vi "TDMS Total Channel Length page.vi"(8 "error in (no error)":errorcluster, 11 "Node Ptr":T1 format="%.0x") -> (0 "error out":errorcluster)   [LabVIEW 2011, in "TDMS Custom Device.lvlib"]
uses:
  TDMS Custom Device.lvlib
  <vilib>/NI Veristand/Custom Device API/Custom Device Item Ref.ctl
  <vilib>/NI Veristand/Custom Device API/Custom Device API.lvlib
panel:
  out "Total Channel Length (elements)":u32
  in  "Header":cluster{"Section Name":string}={"Section Name"="TDMS Mode Channel Settings"}
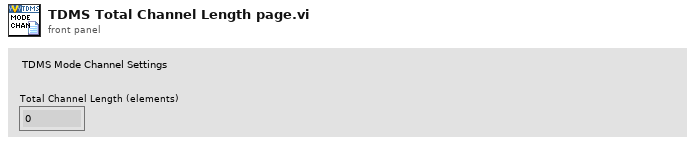
[diagram p1: front panel]
types:
  T1 = typedef "Custom Device API.lvlib/Custom Device Item Ref.ctl" = u64
  T2 = typedef "Custom Device API.lvlib/Custom Device Channel.ctl" = cluster{"Type":T3, "Units":string, "Default Value":dbl, "Faultable":bool, "Scalable":bool}
  T3 = typedef "Custom Device API.lvlib/Custom Device Channel Type.ctl" = enum16{"Input", "Output"}
  T4 = typedef "Custom Device API.lvlib/Custom Device Commands.ctl" = enum16{"Default", "Item renamed", "Shutdown", "Dynamic button pressed"}
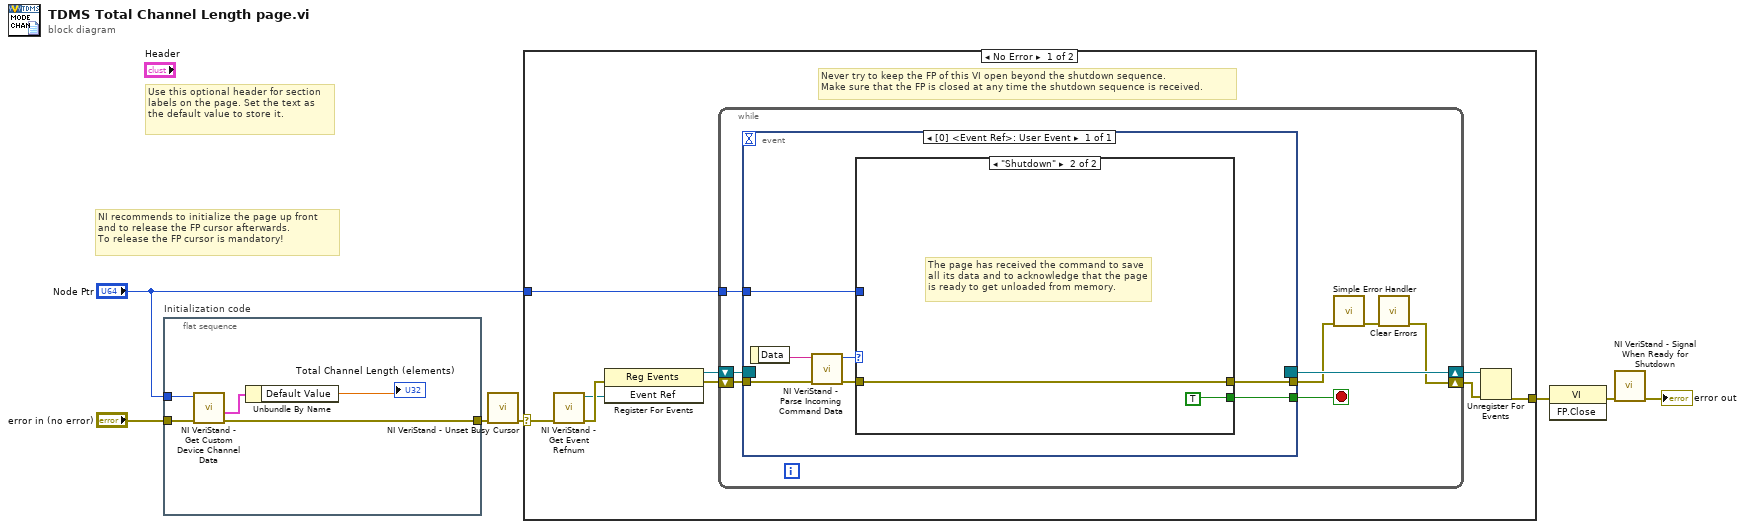
[diagram p0: block diagram]
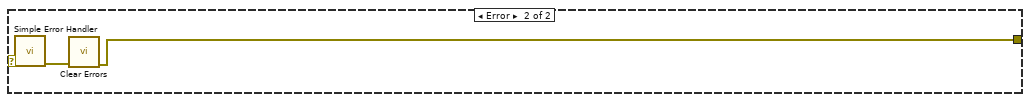
[diagram p3: hidden frame]
diagram:
  # "Use this optional header for section labels on the page. Set the text as the default value to store it."
  # "NI recommends to initialize the page up front\nand to release the FP cursor afterwards.\nTo release the FP cursor is mandatory!"
  n1 = flat-sequence "Initialization code" {
    tunnel: "error in (no error)" -> [w11]
    tunnel: "Node Ptr" -> [w10]
    tunnel: [w9] -> w1
    frame #0 {
      n2 = call <vilib>:"NI VeriStand - Get Custom Device Channel Data.vi"("error in (no error)"=w11, "Channel Ref in"=w10) -> ("error out"=w9:errorcluster, "Channel"=w12:T2)  [unwired: 8 out]
      n3 = Unbundle By Name(w12) -> ("Default Value"=→"Total Channel Length (elements)":dbl)
    }
  }
  n4 = call <vilib>:"NI VeriStand - Unset Busy Cursor.vi"("error in (no error)"=w1) -> ("error out"=w3:errorcluster)  [unwired: 10 out]
  n5 = case shown="No Error" w3 {
    selector: w3 -> [w13 w42]
    tunnel: [w18 w40] -> w7
    tunnel: "Node Ptr" -> [w14 _]
    frame No Error {
      # "Never try to keep the FP of this VI open beyond the shutdown sequence.\nMake sure that the FP is closed at any time the shutdown sequence is received."
      n6 = call <vilib>:"NI VeriStand - Get Event Refnum.vi"("error in (no error)"=w13) -> ("error out"=w21:errorcluster, "Event Ref"=w17:refnum<user-event>)  [unwired: 9 out]
      n7 = register-events(error in=w21, w17) -> (reference out=w15:refnum<event-registration>, error out=w16:errorcluster)  [unwired: 1 in]
      n8 = while {
        tunnel: w14 -> [w25]
        shift-right: [w22] -> w19
        shift-left: w16 -> [w28]
        shift-right: [w29] -> w20
        shift-left: w15 -> [w27]
        stop <- w26 stop-if-true
        n9 = event shown="[0] <Event Ref>: User Event" {
          selector: w27 -> [_]
          dyn-events: [_] -> w29
          timeout: _ -> [_]
          tunnel: w28 -> [w36]
          tunnel: [w32] -> w26
          tunnel: [w31] -> w24
          tunnel: w25 -> [w30]
          event User Event {
            n10 = event-data() -> ("Data"=w35:string)  [unwired: 1 out]
            n11 = call <vilib>:"NI VeriStand - Parse Incoming Command Data.vi"("error in (no error)"=w36, "Incoming data"=w35) -> ("error out"=w34:errorcluster, "Action"=w33:T4)  [unwired: 8 out]
            n12 = case shown="\"Shutdown\"" w33 {
              tunnel: w34 -> [w37 w38]
              tunnel: [_ TRUE] -> w32
              tunnel: [w37 w38] -> w31
              tunnel: w30 -> [_ _]
              frame "Default", Default {
              }
              frame "Shutdown" {
                # "The page has received the command to save all its data and to acknowledge that the page is ready to get unloaded from memory."
              }
            }
          }
        }
        n13 = call <vilib>:"Simple Error Handler.vi"("error in (no error)"=w24) -> ("error out"=w23:errorcluster)  [unwired: 1 in, 7 out]
        n14 = call <vilib>:"Clear Errors.vi"("error in (no error)"=w23) -> ("error out"=w22:errorcluster)  [unwired: 6 out]
      }
      n15 = Unregister For Events(event registration refnum=w20, error in=w19) -> (error out=w18:errorcluster)
    }
    frame Error {
      n16 = call <vilib>:"Simple Error Handler.vi"("error in (no error)"=w42) -> ("error out"=w41:errorcluster)  [unwired: 1 in, 7 out]
      n17 = call <vilib>:"Clear Errors.vi"("error in (no error)"=w41) -> ("error out"=w40:errorcluster)  [unwired: 6 out]
    }
  }
  n18 = invoke class="VI" method="FP.Close"(error in=w7) -> (error out=w6:errorcluster)  [unwired: 2 in, 2 out]
  n19 = call <vilib>:"NI VeriStand - Signal When Ready for Shutdown.vi"("error in (no error)"=w6) -> ("error out"=→"error out":errorcluster)  [unwired: 10 out]
